vi "Release Semaphore.vi"(8 "error in (no error)":errorcluster, 11 "Serial IO in":refnum<class "Serial IO.lvclass">) -> (0 "error out":errorcluster, 3 "Serial IO out":refnum<class "Serial IO.lvclass">)   [LabVIEW 2015, in "Serial IO.lvclass"]
doc: "Release the semaphore acquired to prevent serial port clashes in the program."
uses:
  Serial IO.lvclass
  Serial IO.lvclass/Serial IO.ctl
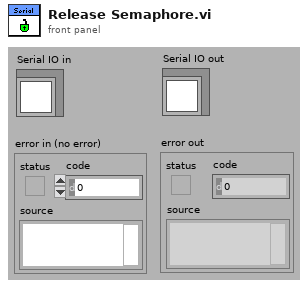
[diagram p1: front panel]
types:
  T1 = typedef "Semaphore RefNum" = refnum<k1>
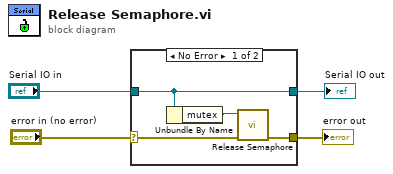
[diagram p0: block diagram]
diagram:
  n1 = case shown="No Error" "error in (no error)" {
    selector: "error in (no error)" -> [w7 w10]
    tunnel: [w6 w10] -> w3
    tunnel: [w5 w9] -> w1
    tunnel: "Serial IO in" -> [w5 w9]
    frame No Error {
      n2 = Unbundle By Name(w5) -> ("mutex"=w8:T1)
      n3 = call <vilib>:"Release Semaphore.vi"("error in (no error)"=w7, "semaphore"=w8) -> ("error out"=w6:errorcluster)  [unwired: 4 in, 1 out]
    }
    frame Error {
    }
  }
  "error out" <- w3
  "Serial IO out" <- w1
